vi "05. Native MQTT Service Client.vi"() -> ()   [LabVIEW 2019]
uses:
  Actor/Response -- cluster.ctl
  <vilib>/LabVIEW Open Source Project/MQTT Control Packets/Control Packets/ControlPacket/ControlPacket.lvclass/ControlPacket.ctl
  eb8eb180-2280-4b70-97f6-c873bf82b039.vi
  b06ea2ed-6302-4e94-bd79-5b3576c24717.vi
  <vilib>/LabVIEW Open Source Project/MQTT Control Packets/Control Packets/PUBLISH/PUBLISH.lvclass
  C:/Program Files (x86)/National Instruments/LabVIEW 2019/vi.lib/LabVIEW Open Source Project/MQTT Control Packets/Control Packets/ControlPacket/ControlPacket.lvclass
  <vilib>/JDP Science/JSONtext/JSON text to Variant.vi
  <vilib>/JDP Science/JSONtext/LVClass Serializer/JSONtext LVClass Serializer.lvclass
  <vilib>/LabVIEW Open Source Project/MQTT Control Packets/Control Packets/ControlPacket/ControlPacket.lvclass
  <vilib>/JDP Science/JSONtext/JSONtext.lvlib
panel:
  in  "parameters 2":string
  out "Value":dbl
  in  "Service Namespace":string="demo/router"
  out "Topic":string
  out "<JSON>Response":string
  in  "parameters":string="{\"test\": \"string\"}"
  in  "Method":string
  in  "Send Req":bool
  in  "Get Value":bool
  in  "Echo":bool
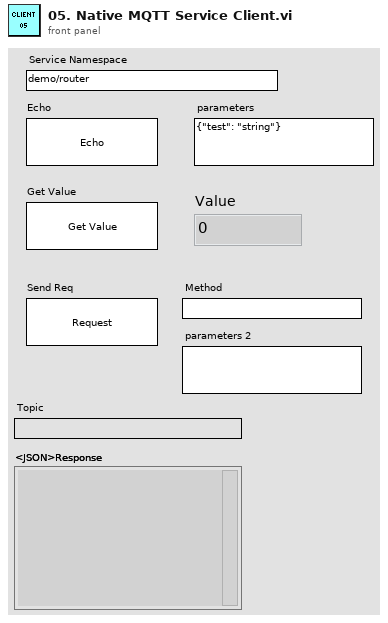
[diagram p1: front panel]
types:
  T1 = typedef "Actor Private Data.ctl" = cluster{"Client":refnum<class "Client.lvclass">, "QualifiedName":string, "EventReg":refnum<event-registration>, "Private Events":T2}
  T2 = typedef "Actor Private Events -- cluster.ctl" = cluster{"Stop":refnum<user-event>, "Subscribe":refnum<user-event>, "Unsubscribe":refnum<user-event>, "publish":refnum<user-event>}
  T3 = typedef "Response -- cluster.ctl" = cluster{"<JSON>result":string, "id":string, "<JSON>error":string}
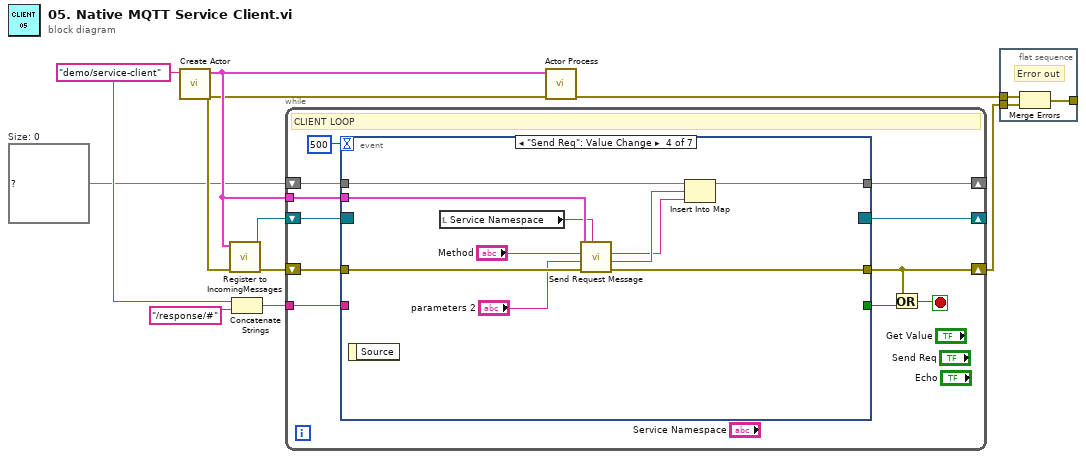
[diagram p0: block diagram]
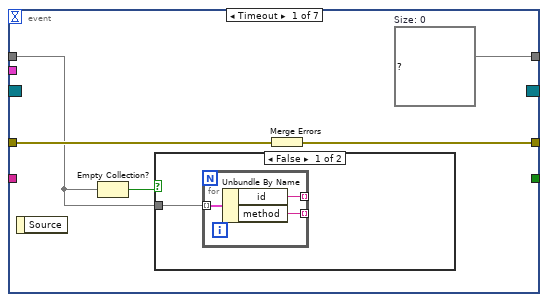
[diagram p2: hidden frame]
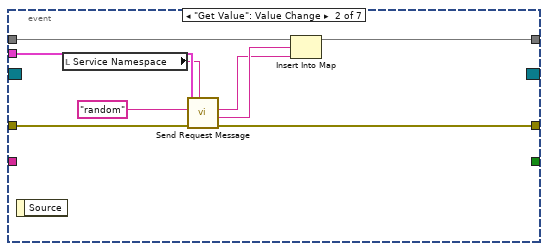
[diagram p4: hidden frame]
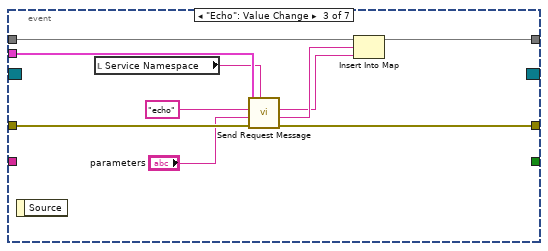
[diagram p5: hidden frame]
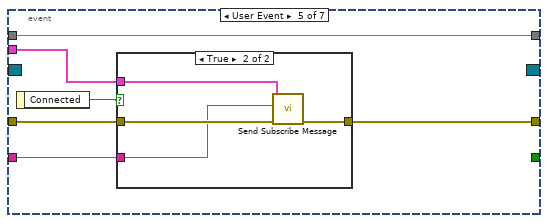
[diagram p6: hidden frame]
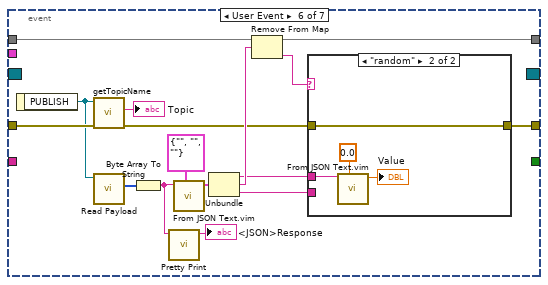
[diagram p8: hidden frame]
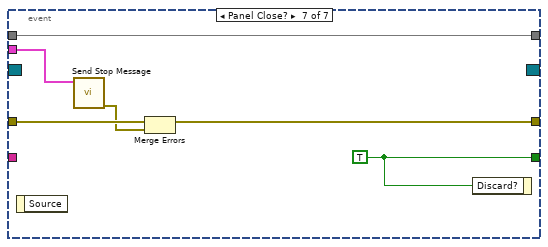
[diagram p10: hidden frame]
diagram:
  w1 = map{string, string} {}  # Size: 0
  w4 = "demo/service-client" ("QualifiedName")
  n1 = call "Create Actor.vi"("QualifiedName"=w4) -> ("error out"=w5:errorcluster, "Actor Class"=w9:T1)  [unwired: 9 in]
  n2 = call "Register to IncomingMessages.vi"("error in"=w5, "Actor Class"=w9) -> ("error out"=w8:errorcluster, "Incoming Messages"=w10:refnum<event-registration>)  [unwired: 8 in]
  n3 = Concatenate Strings(w4, "/response/#" ("QualifiedName")) -> (w2:string)
  n4 = while {
    tunnel: w9 -> [w19]
    shift-right: [w16] -> _
    shift-left: w10 -> [w17]
    shift-right: [w14] -> w7
    shift-left: w8 -> [w15]
    tunnel: w2 -> [w13]
    shift-right: [w11] -> _
    shift-left: w1 -> [w12]
    stop <- w20 stop-if-true
    # "CLIENT LOOP"
    n5 = event shown="[3] \"Send Req\": Value Change" {
      selector: w17 -> [_ _ _ _ _ _ _]
      dyn-events: [_ _ _ _ _ _ _] -> w16
      timeout: 500 -> [_ _ _ _ _ _ _]
      tunnel: [_ _ _ _ _ _ w97] -> w21
      tunnel: w19 -> [_ w37 w47 w57 w63 _ w96]
      tunnel: [w25 w38 w48 w58 w64 w71 w93] -> w14
      tunnel: w15 -> [w26 w39 w49 w59 w65 w86 w95]
      tunnel: w13 -> [_ _ _ _ w61 _ _]
      tunnel: w12 -> [w23 w34 w43 w54 w60 w78 w92]
      tunnel: [w24 w31 w40 w51 w60 w74 w92] -> w11
      event Timeout {
        w24 = map{string, string} {}  # Size: 0
        n6 = event-data() -> ()  [unwired: 1 in, 1 out]
        n7 = Empty Collection?(1:w23) -> (0:w22:bool)
        n8 = case shown="False" w22 {
          tunnel: w23 -> [w27 _]
          frame False {
            n9 = for {
              tunnel: w27 -> [w30] mode=indexing
              tunnel: [w29] -> _ mode=indexing
              tunnel: [w28] -> _ mode=indexing
              n10 = Unbundle By Name(w30) -> ("id"=w29:string, "method"=w28:string)
            }
          }
          frame True {
          }
        }
        n11 = Merge Errors(w26) -> (w25:errorcluster)
      }
      event "Get Value": Value Change {
        n12 = event-data() -> ()  [unwired: 1 in, 1 out]
        n13 = local read "Service Namespace"() -> (w35:string)
        n14 = call "Send Request Message.vi"("Qualified Name"=w35, "error in"=w39, "method"="random", "Actor Class"=w37) -> ("error out"=w38:errorcluster, "id out"=w33:string, "method dup"=w32:string)  [unwired: 5 in]
        n15 = Insert Into Map(map in=w34, key=w33, value=w32) -> (map out=w31:map{string, string})  [unwired: 2 out]
      }
      event "Echo": Value Change {
        n16 = event-data() -> ()  [unwired: 1 in, 1 out]
        n17 = local read "Service Namespace"() -> (w44:string)
        n18 = call "Send Request Message.vi"("Qualified Name"=w44, "error in"=w49, "<JSON>params"="parameters", "method"="echo", "Actor Class"=w47) -> ("error out"=w48:errorcluster, "id out"=w42:string, "method dup"=w41:string)  [unwired: 4 in]
        n19 = Insert Into Map(map in=w43, key=w42, value=w41) -> (map out=w40:map{string, string})  [unwired: 2 out]
      }
      event "Send Req": Value Change {
        n20 = event-data() -> ()  [unwired: 1 in, 1 out]
        n21 = local read "Service Namespace"() -> (w55:string)
        n22 = call "Send Request Message.vi"("Qualified Name"=w55, "error in"=w59, "<JSON>params"="parameters 2", "method"="Method", "Actor Class"=w57) -> ("error out"=w58:errorcluster, "id out"=w53:string, "method dup"=w52:string)  [unwired: 4 in]
        n23 = Insert Into Map(map in=w54, key=w53, value=w52) -> (map out=w51:map{string, string})  [unwired: 2 out]
      }
      event User Event {
        n24 = event-data() -> ("Connected"=w62:bool)  [unwired: 1 in]
        n25 = case shown="True" w62 {
          tunnel: w65 -> [w66 w70]
          tunnel: [w66 w69] -> w64
          tunnel: w63 -> [_ w68]
          tunnel: w61 -> [_ w67]
          frame False {
          }
          frame True {
            n26 = call "Send Subscribe Message.vi"("error in"=w70, "Topic"=w67, "Actor Class"=w68) -> ("error out"=w69:errorcluster)  [unwired: 8 in]
          }
        }
      }
      event User Event {
        n27 = event-data() -> ("PUBLISH"=w85:refnum<class "PUBLISH.lvclass">)  [unwired: 1 in]
        n28 = call <vilib>:"getTopicName.vi"("error in (no error)"=w86, "PUBLISH in"=w85) -> ("error out"=w72:errorcluster, "Topic"=→"Topic":string)  [unwired: 7 in, 1 out]
        n29 = call <vilib>:"Read Payload.vi"("ControlPacket in"=w85) -> ("Payload"=w84:u8[])  [unwired: 9 in, 1 out]
        n30 = Byte Array To String(unsigned byte array=w84) -> (string=w81:string)
        n31 = call <vilib>:"Pretty Print.vi"("JSON"=w81) -> ("<JSON>"=→"<JSON>Response":string)  [unwired: 8 in, 2 out]
        n32 = call "From JSON Text.vim"("Data Type and Default Value"=T3 {"<JSON>result"="", "id"="", "<JSON>error"=""} ("response"), "JSON"=w81) -> ("Data out"=w79:T3)  [unwired: 8 in, 1 out]
        n33 = Unbundle(w79) -> ("<JSON>result"=w76:string, "id"=w77:string, "<JSON>error"=w75:string)
        n34 = Remove From Map(10:w77, 11:w78) -> (1:w73:string, 3:w74:map{string, string})  [unwired: 1 out]
        n35 = case shown="\"random\"" w73 {
          tunnel: w76 -> [_ w89]
          tunnel: w75 -> [_ _]
          tunnel: w72 -> [w87 w91]
          tunnel: [w87 w91] -> w71
          frame Default {
          }
          frame "random" {
            n36 = call "From JSON Text.vim"("Data Type and Default Value"=0.0, "JSON"=w89) -> ("Data out"=→"Value":dbl)  [unwired: 8 in, 1 out]
          }
        }
      }
      event Panel Close? {
        w97 = TRUE ("Discard?")
        n37 = event-data() -> ()  [unwired: 1 in, 1 out]
        n38 = call "Send Stop Message.vi"("Actor Class"=w96) -> ("error out"=w94:errorcluster)  [unwired: 10 in]
        n39 = Merge Errors(w95, w94) -> (w93:errorcluster)
        n40 = event-data("Discard?"=w97) -> ()  [unwired: 1 in, 1 out]
      }
    }
    n41 = Or(x=w14, y=w21) -> (x .or. y?=w20:bool)
  }
  n42 = call "Actor Process.vi"("error in"=w5, "Actor Class"=w9) -> ("error out"=w6:errorcluster)  [unwired: 9 in]
  n43 = flat-sequence {
    tunnel: w6 -> [w100]
    tunnel: w7 -> [w99]
    tunnel: [w98] -> _
    frame #0 {
      # "Error out"
      n44 = Merge Errors(w100, w99) -> (w98:errorcluster)
    }
  }
